vi "GPSDO HP5335A CrossReference.vi"() -> ()   [LabVIEW 2015]
panel:
  out "Measurment":ext format="%.9e"
  out "Line":string
  out "Measurement":cluster{"Measurment":ext, "Measurment":ext}(graph)
  out "error out":errorcluster
  in  "Stop Button":bool
  in  "AC\nDC 2":bool
  in  "AC\nDC":bool
  in  "Gate Delay":ext=0.25 format="%.3f"
  in  "error in":errorcluster
  in  "Path":path
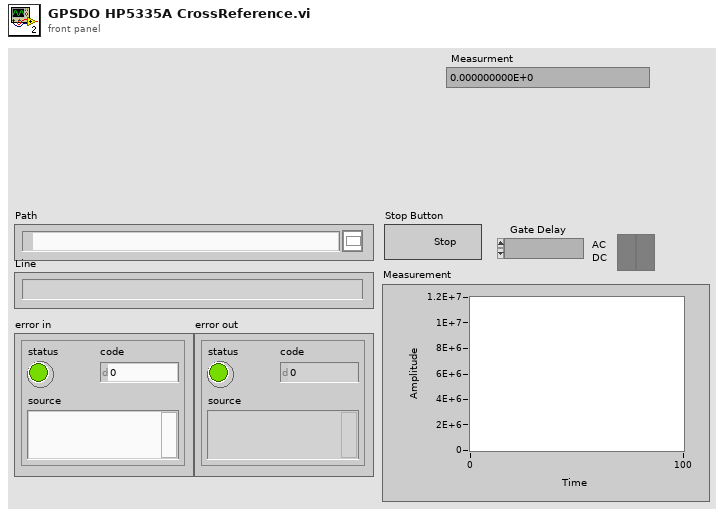
[diagram p1: front panel]
types:
  T1 = enum16{"open", "replace", "create", "open or create", "replace or create", "replace or create with confirmation"}
  T2 = typedef "LVDateTimeRec.ctl" = cluster{"fractional second":dbl, "second":i32, "minute":i32, "hour":i32, "day of month":i32, "month":i32, "year":i32, "day of week":i32, "day of year":i32, "DST":i32}
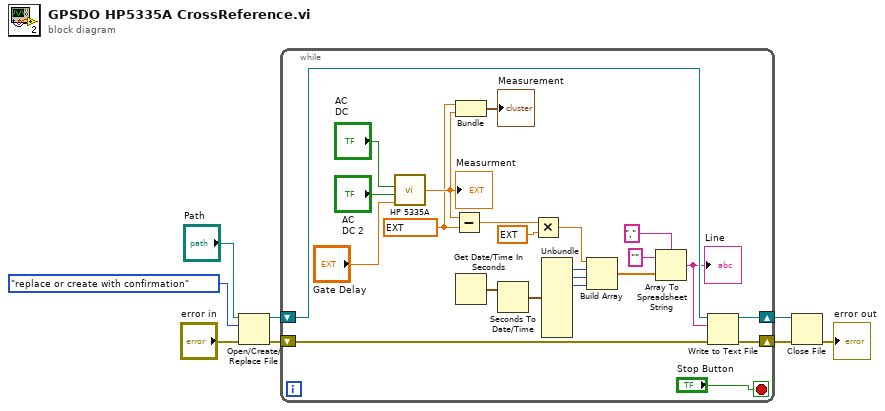
[diagram p0: block diagram]
diagram:
  n1 = Open/Create/Replace File(file path (use dialog)="Path", error in="error in", operation (0:open)=T1."replace or create with confirmation") -> (refnum out=w6:refnum<file>, error out=w5:errorcluster)  [unwired: 3 in, 1 out]
  n2 = while {
    shift-right: [w26] -> w3
    shift-left: w6 -> [w29]
    shift-right: [w27] -> w4
    shift-left: w5 -> [w28]
    stop <- "Stop Button" stop-if-true
    w12 = ext 10000000.0 ("Measurment")
    n3 = call <instrlib>:"HP 5335A.vi"("Gate Delay"="Gate Delay", 2:"AC\nDC"="AC\nDC 2", 3:"AC\nDC"="AC\nDC") -> ("Measurment"=w13:ext)  [unwired: 1 in]
    "Measurment" <- w13
    n4 = Subtract(x=w13, y=w12) -> (x-y=w11:ext)
    n5 = Bundle("Measurment"=w12, "Measurment"=w13) -> (→"Measurement":cluster{"Measurment":ext, "Measurment":ext})  [unwired: 1 in]
    n6 = Get Date/Time In Seconds() -> (seconds since 1Jan1904=w31:timestamp)
    n7 = Seconds To Date/Time(time stamp (now)=w31) -> (date time rec=w30:T2)  [unwired: 1 in]
    n8 = Multiply(x=w11, y=ext 1000.0) -> (x*y=w10:ext)
    n9 = Unbundle(w30) -> ("second"=w25:i32, "minute"=w24:i32, "hour"=w23:i32)  [unwired: 7 out]
    n10 = Build Array(w10, w25, w24, w23) -> (w22:ext[])
    n11 = Array To Spreadsheet String(delimiter (Tab)=",", array=w22, 3:"" ("format string")) -> (spreadsheet string=w19:string)
    "Line" <- w19
    n12 = Write to Text File(file (use dialog)=w29, text=w19, error in=w28) -> (refnum out=w26:refnum<file>, error out=w27:errorcluster)  [unwired: 1 in, 1 out]
  }
  n13 = Close File(refnum=w3, error in=w4) -> (error out=→"error out":errorcluster)  [unwired: 1 out]
